vi "Part 1.vi"(11 "Input":string) -> (3 "Output":i64)   [LabVIEW 2021]
uses:
  <userlib>/_OpenG.lib/string/string.llb/Convert EOLs (String)__ogtk.vi
panel:
  out "Array 2":T1(array[cluster])
  out "Array":bool[](array[boolean])
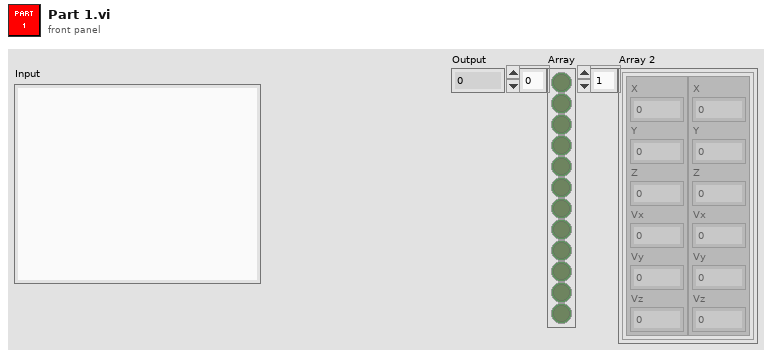
[diagram p1: front panel]
types:
  T1 = cluster{cluster{"X":ext, "Y":ext, "Z":ext, "Vx":ext, "Vy":ext, "Vz":ext}, cluster{"X":ext, "Y":ext, "Z":ext, "Vx":ext, "Vy":ext, "Vz":ext}}[]
  T2 = cluster{"X":ext, "Y":ext, "Z":ext, "Vx":ext, "Vy":ext, "Vz":ext}
  T3 = cluster{"X":ext, "Y":ext, "Z":ext, "Vx":ext, "Vy":ext, "Vz":ext}[]
  T4 = cluster{cluster{"X":ext, "Y":ext, "Z":ext, "Vx":ext, "Vy":ext, "Vz":ext}, cluster{"X":ext, "Y":ext, "Z":ext, "Vx":ext, "Vy":ext, "Vz":ext}}
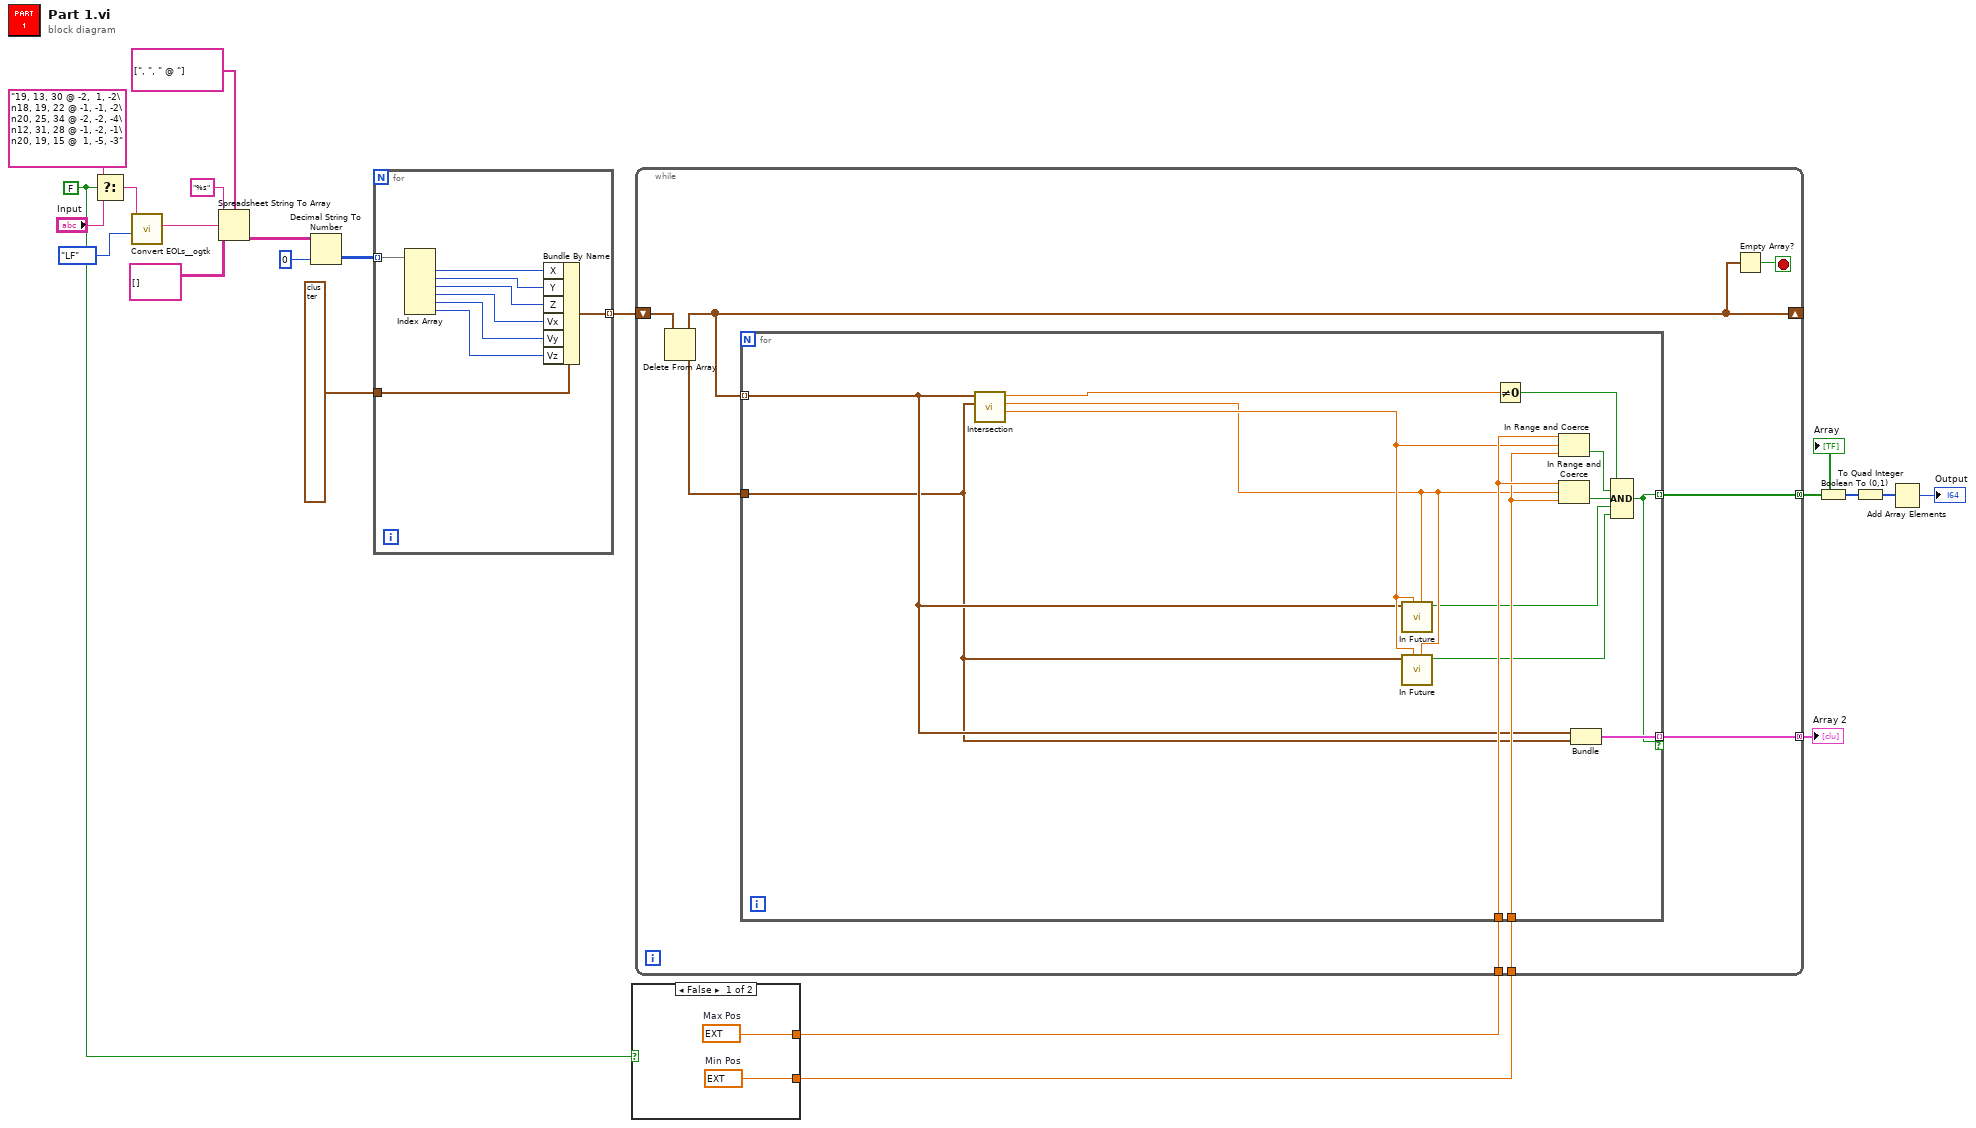
[diagram p0: block diagram]
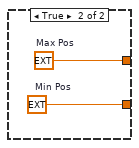
[diagram p2: hidden frame]
diagram:
  w1 = FALSE
  n1 = Select(t="19, 13, 30 @ -2,  1, -2\n18, 19, 22 @ -1, -1, -2\n20, 25, 34 @ -2, -2, -4\n12, 31, 28 @ -1, -2, -1\n20, 19, 15 @  1, -5, -3", s=w1, f="Input") -> (s? t:f=w15:string)
  n2 = call-poly <userlib>:"Convert EOLs__ogtk.vi"("Convert to:"=enum16{"CR", "LF", "CRLF"}."LF", "String in"=w15) -> ("String out"=w19:string)  [unwired: 9 in]
  n3 = Spreadsheet String To Array(delimiter (Tab)=string[] [", ", " @ "], format string="%s", spreadsheet string=w19, array type (2D Dbl)=string[][] []) -> (array=w13:string[][])
  n4 = Decimal String To Number(string=w13, default (0L)=i64 0) -> (number=w11:i64[][])  [unwired: 1 in, 1 out]
  n5 = for {
    tunnel: w11 -> [w30] mode=indexing
    tunnel: T2 {"X"=0.0, "Y"=0.0, "Z"=0.0, "Vx"=0.0, "Vy"=0.0, "Vz"=0.0} -> [w29]
    tunnel: [w28] -> w9 mode=indexing
    n6 = Index Array(array=w30) -> (element #1=w27:i64, element #2=w26:i64, element #3=w25:i64, element #4=w24:i64, element #5=w23:i64, element #6=w22:i64)  [unwired: 6 in]
    n7 = Bundle By Name(cluster=w29, "X"=w27, "Y"=w26, "Z"=w25, "Vx"=w24, "Vy"=w23, "Vz"=w22) -> (w28:T2)
  }
  n8 = case shown="False" w1 {
    tunnel: [w32 w34] -> w4
    tunnel: [w31 w33] -> w3
    frame False {
      w31 = ext 200000000000000.0  # Min Pos
      w32 = ext 400000000000000.0  # Max Pos
    }
    frame True {
      w34 = ext 27.0  # Max Pos
      w33 = ext 7.0  # Min Pos
    }
  }
  n9 = while {
    shift-right: [w40] -> _
    shift-left: w9 -> [w42]
    tunnel: [w38] -> w8 mode=concatenating
    tunnel: w4 -> [w37]
    tunnel: w3 -> [w36]
    tunnel: [w35] -> w2 mode=concatenating
    stop <- w41 stop-if-true
    n10 = Delete From Array(array=w42) -> (deleted portion=w39:T2, array with subset deleted=w40:T3)  [unwired: 2 in]
    n11 = for {
      tunnel: w40 -> [w46] mode=indexing
      tunnel: w39 -> [w43]
      tunnel: [w44] -> w38 mode=indexing
      tunnel: w37 -> [w56]
      tunnel: w36 -> [w55]
      tunnel: [w45] -> w35 mode=indexing if=w44
      n12 = call "Intersection.vi"("Line2"=w43, "Line1"=w46) -> ("Px"=w50:dbl, "Py"=w49:dbl, "denom"=w53:dbl)  [unwired: 7 in]
      n13 = call "In Future.vi"("Py"=w49, "Px"=w50, "Line"=w46) -> ("Future?"=w48:bool)  [unwired: 8 in]
      n14 = call "In Future.vi"("Py"=w49, "Px"=w50, "Line"=w43) -> ("Future?"=w47:bool)  [unwired: 8 in]
      n15 = Not Equal To 0?(x=w53) -> (x != 0?=w51:bool)
      n16 = In Range and Coerce(upper limit=w56, x=w50, lower limit=w55) -> (In Range?=w52:bool)  [unwired: 1 out]
      n17 = In Range and Coerce(upper limit=w56, x=w49, lower limit=w55) -> (In Range?=w54:bool)  [unwired: 1 out]
      n18 = Bundle(w46, w43) -> (w45:T4)  [unwired: 1 in]
      n19 = Compound Arithmetic op=AND(w51, w52, w54, w48, w47) -> (w44:bool)
    }
    n20 = Empty Array?(array=w40) -> (empty?=w41:bool)
  }
  "Array" <- w8
  "Array 2" <- w2
  n21 = Boolean To (0,1)(Boolean=w8) -> (0, 1=w7:i16[])
  n22 = To Quad Integer(1:w7) -> (0:w6:i64[])
  n23 = Add Array Elements(numeric array=w6) -> (sum=→"Output":i64)
